vi "MotorTest.vi"() -> ()   [LabVIEW 2015]
panel:
  in  "error in (no error)":errorcluster
  out "CoverState":enum16{"In", "Moving", "Out", "Wait"}(ring)
  in  "Out limit":bool
  in  "In limit":bool
  in  "stop":bool
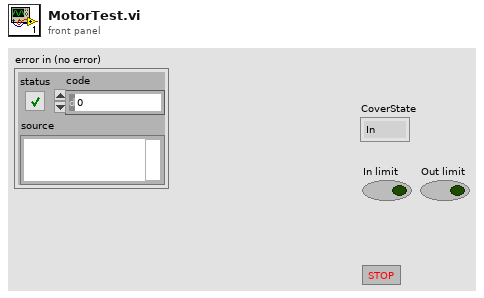
[diagram p1: front panel]
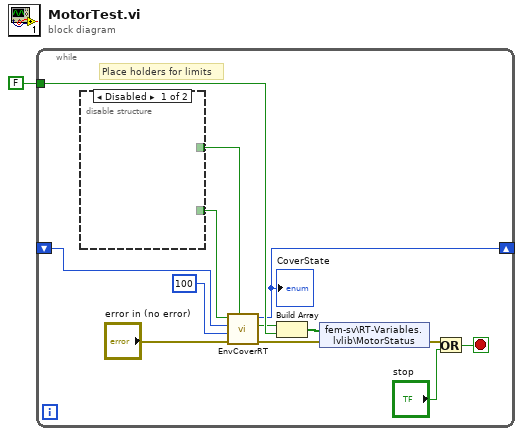
[diagram p0: block diagram]
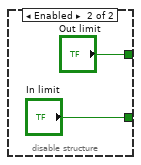
[diagram p2: hidden frame]
diagram:
  n1 = while {
    shift-right: [w2] -> _
    shift-left: _ -> [w12]
    tunnel: FALSE -> [w7]
    stop <- w13 stop-if-true
    # "Place holders for limits"
    n2 = disable-structure shown="Disabled" {
      disable-tunnel: [_ "In limit"] -> w9
      disable-tunnel: [_ "Out limit"] -> w8
      frame Disabled {
      }
      frame Enabled {
      }
    }
    n3 = call "EnvCoverRT.vi"("Out limit"=w8, "error in (no error)"="error in (no error)", "ms timeout (0)"=100, "Status in"=w12, "In limit"=w9) -> ("error out"=w4:errorcluster, "Ready?"=w6:bool, "Status out"=w2:enum16{"In", "Moving", "Out", "Wait"})  [unwired: 4 in]
    "CoverState" <- w2
    n4 = Build Array(w6, w7) -> (w5:bool[])
    n5 = shared-variable "fem-sv\\RT-Variables.lvlib\\MotorStatus"(w5, error in=w4) -> (error out=w3:errorcluster)
    n6 = Or(x=w3, y="stop") -> (x .or. y?=w13:bool)
  }
